vi "Train ramp.vi"(7 "pwr supply in":refnum<class "Power Supply.lvclass">, 9 "input":dbl[unit], 11 "field":dbl[unit]) -> (0 "output":dbl[unit], 2 "change?":bool, 3 "pwr supply out":refnum<class "Power Supply.lvclass">)   [LabVIEW 2009, in "Power Supply.lvclass"]
uses:
  Power Supply.lvclass
  Power Supply.lvclass/Power Supply.ctl
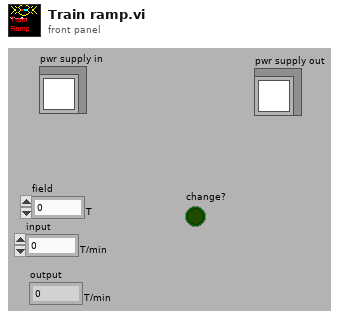
[diagram p1: front panel]
types:
  T1 = cluster{"Training Field":dbl[unit][], "Training Speed":dbl[unit][]}
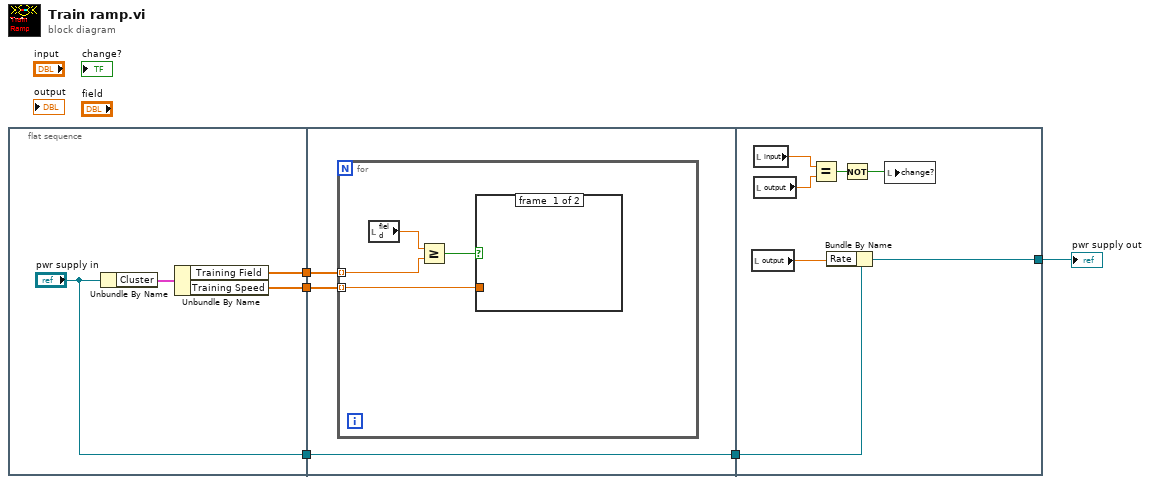
[diagram p0: block diagram]
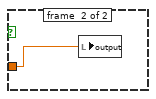
[diagram p2: hidden frame]
diagram:
  n1 = flat-sequence {
    tunnel: [w8] -> w5
    tunnel: [w7] -> w4
    tunnel: ["pwr supply in"] -> w3
    tunnel: w5 -> [w12]
    tunnel: w4 -> [w11]
    tunnel: w3 -> [w10]
    tunnel: [w10] -> w2
    tunnel: w2 -> [w24]
    tunnel: [w22] -> w1
    frame #0 {
      n2 = Unbundle By Name("pwr supply in") -> ("Cluster"=w9:T1)
      n3 = Unbundle By Name(w9) -> ("Training Field"=w8:dbl[unit][], "Training Speed"=w7:dbl[unit][])
    }
    frame #1 {
      n4 = for {
        tunnel: w12 -> [w15] mode=indexing
        tunnel: w11 -> [w13] mode=indexing
        n5 = local read "field"() -> (w16:dbl[unit])
        n6 = Greater Or Equal?(x=w16, y=w15) -> (x >= y?=w14:bool)
        n7 = case shown="True" w14 {
          tunnel: w13 -> [_ w17]
          frame #0 {
          }
          frame #1 {
            n8 = local write "output"(w17) -> ()
          }
        }
      }
    }
    frame #2 {
      n9 = local read "output"() -> (w23:dbl[unit])
      n10 = local read "input"() -> (w21:dbl[unit])
      n11 = local read "output"() -> (w20:dbl[unit])
      n12 = Equal?(x=w21, y=w20) -> (x = y?=w19:bool)
      n13 = Bundle By Name(cluster=w24, "Rate"=w23) -> (w22:refnum<class "Power Supply.lvclass">)
      n14 = Not(x=w19) -> (.not. x?=w18:bool)
      n15 = local write "change?"(w18) -> ()
    }
  }
  "pwr supply out" <- w1
